vi "betweenLimitsIndex.vi"(9 "upper limit":dbl=0.01 format="%#_13g", 10 "lower limit":dbl=0.007 format="%#_13g", 11 "Data":dbl[](array[numeric])) -> (3 "index":i32[](array[numeric]))   [LabVIEW 2017]
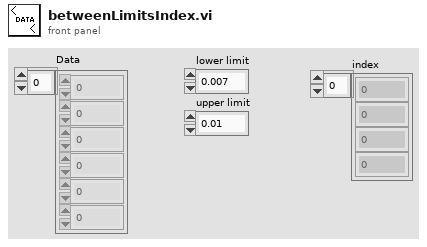
[diagram p1: front panel]
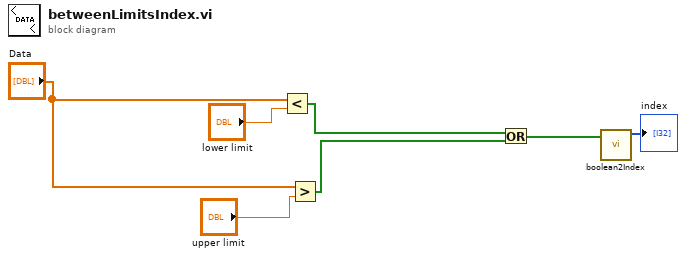
[diagram p0: block diagram]
diagram:
  n1 = Less?(x="Data", y="lower limit") -> (x < y?=w4:bool[])
  n2 = Greater?(x="Data", y="upper limit") -> (0:w3:bool[])
  n3 = Or(x=w4, y=w3) -> (x .or. y?=w2:bool[])
  n4 = call "boolean2Index.vi"("boolean"=w2) -> ("index"=→"index":i32[])  [unwired: 10 in]
